vi "Configure System (Display).vi"(7 "Display Enable (T:Enable)":bool=TRUE, 8 "error in (no error)":errorcluster, 9 "User Comment (\"\")":string, 10 "Display Page (0: MEAS)":u16(ring) items=["Measurement Display", "BIN No. Display", "BIN Count Display", "List Sweep Display", "Measurement Setup", "Correction Setup", "Limit Table Setup", "List Sweep Setup", "Catalog", "System Information", "Self Test", "Large Display", "System Configuration", "Service"], 11 "VISA resource name":refnum<visa-resource-name>) -> (0 "error out":errorcluster, 3 "VISA resource name out":refnum<visa-resource-name>)   [LabVIEW 2017, in "Agilent E4980.lvlib"]
doc: "Enables or disables display updates of the screen, selects the display page, and sets comments."
uses:
  Agilent E4980.lvlib
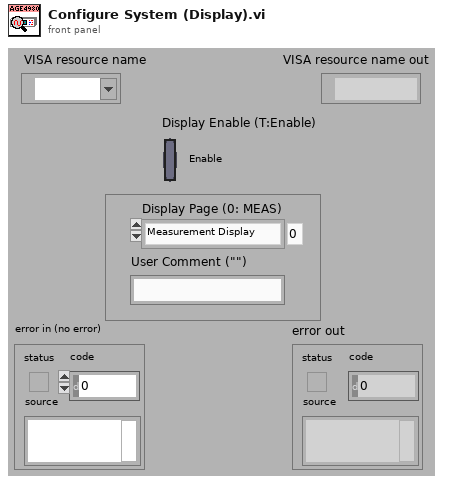
[diagram p1: front panel]
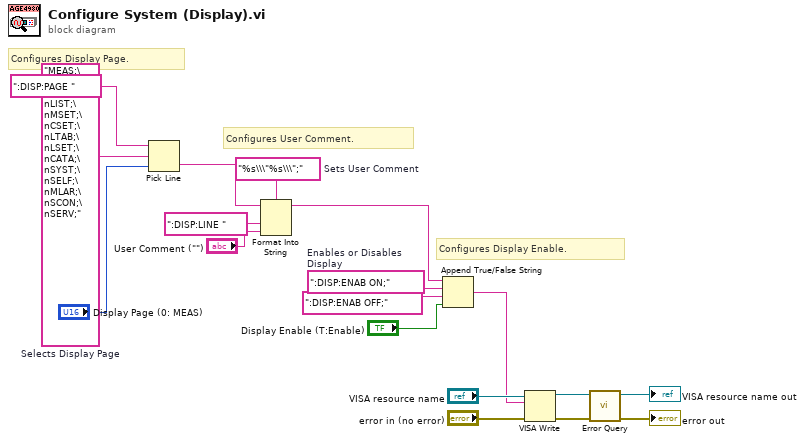
[diagram p0: block diagram]
diagram:
  w12 = "%s\\\"%s\\\";"  # Sets User Comment
  w14 = "MEAS;\nBNUM;\nBCO;\nLIST;\nMSET;\nCSET;\nLTAB;\nLSET;\nCATA;\nSYST;\nSELF;\nMLAR;\nSCON;\nSERV;"  # Selects Display Page
  w18 = ":DISP:ENAB ON;"  # Enables or Disables Display
  # "Configures Display Page."
  # "Configures User Comment."
  # "Configures Display Enable."
  n1 = Pick Line(string ("")=":DISP:PAGE ", multi-line string=w14, line index="Display Page (0: MEAS)") -> (output string=w13:string)
  n2 = Format Into String(format string=w12, initial string=w13, ":DISP:LINE ", "User Comment (\"\")") -> (resulting string=w2:string)  [unwired: 1 in, 1 out]
  n3 = Append True/False String(1:"Display Enable (T:Enable)", 2:":DISP:ENAB OFF;" ("true string"), 3:w18, 4:w2) -> (0:w1:string)
  n4 = VISA Write(VISA resource name="VISA resource name", write buffer=w1, error in (no error)="error in (no error)") -> (VISA resource name out=w7:refnum<visa-resource-name>, error out=w6:errorcluster)  [unwired: 1 out]
  n5 = call "Error Query.vi"("error in (no error)"=w6, "VISA resource name"=w7) -> ("error out"=→"error out":errorcluster, "VISA resource name out"=→"VISA resource name out":refnum<visa-resource-name>)  [unwired: 6 in, 2 out]
